vi "4155C PulsedStressV Config SMUs v2.0.vi"(0 "VISA resource name in":refnum<visa-resource-name>, 1 "Pulse period":dbl=0.05 min=0.005 max=1.0 step=0.0001 format="%.4f", 2 "Pulsed Stress V - Source/Common":u32(ring) items=["SMU1  ", "SMU2  ", "SMU3  ", "SMU4  ", "SMU5  ", "SMU6  "], 3 "Pulse width":dbl=0.0005 min=0.0005 max=0.1 step=0.0001 format="%.4f", 4 "Pulsed Stress V - Drain":u32(ring)=1 items=["SMU1  ", "SMU2  ", "SMU3  ", "SMU4  ", "SMU5  ", "SMU6  "], 5 "error in (no error)":errorcluster, 6 "Gate ON voltage":dbl min=-100.0 max=100.0 step=0.005 format="%.3f", 7 "Drain Voltage":dbl min=-100.0 max=100.0 step=0.005 format="%.3f", 8 "Pulsed Stress V - Gate":u32(ring)=2 items=["SMU1  ", "SMU2  ", "SMU3  ", "SMU4  ", "SMU5  ", "SMU6  "], 9 "Pulsed Stress V - Vextra":u32(ring)=1 items=["VSU1  ", "VSU2  "], 10 "Pulsed Stress V - Probe 4":u32(ring)=3 items=["SMU1  ", "SMU2  ", "SMU3  ", "SMU4  ", "SMU5  ", "SMU6  "], 12 "Gate Standby":bool, 13 "Drain Standby":bool, 15 "Probe 4":cluster{"on/off":bool, "Voltage":dbl} {"Voltage" min=-100.0 max=100.0 format="%.2f"}, 17 "Base voltage":dbl format="%^.4e") -> (14 "VISA Resource Name out":refnum<visa-resource-name>, 19 "error out":errorcluster)   [LabVIEW 2016]
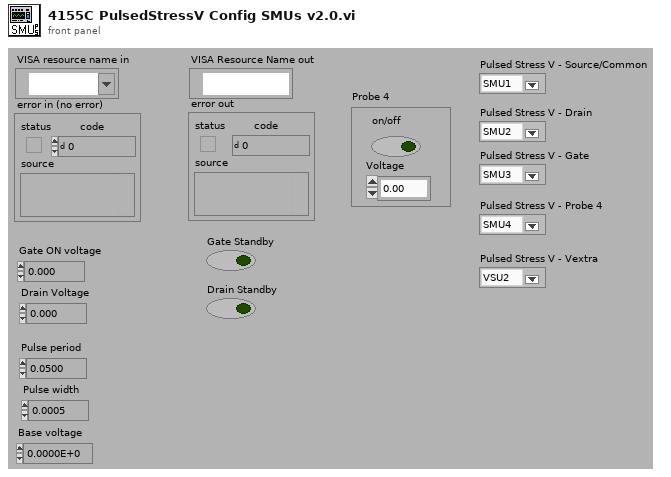
[diagram p1: front panel]
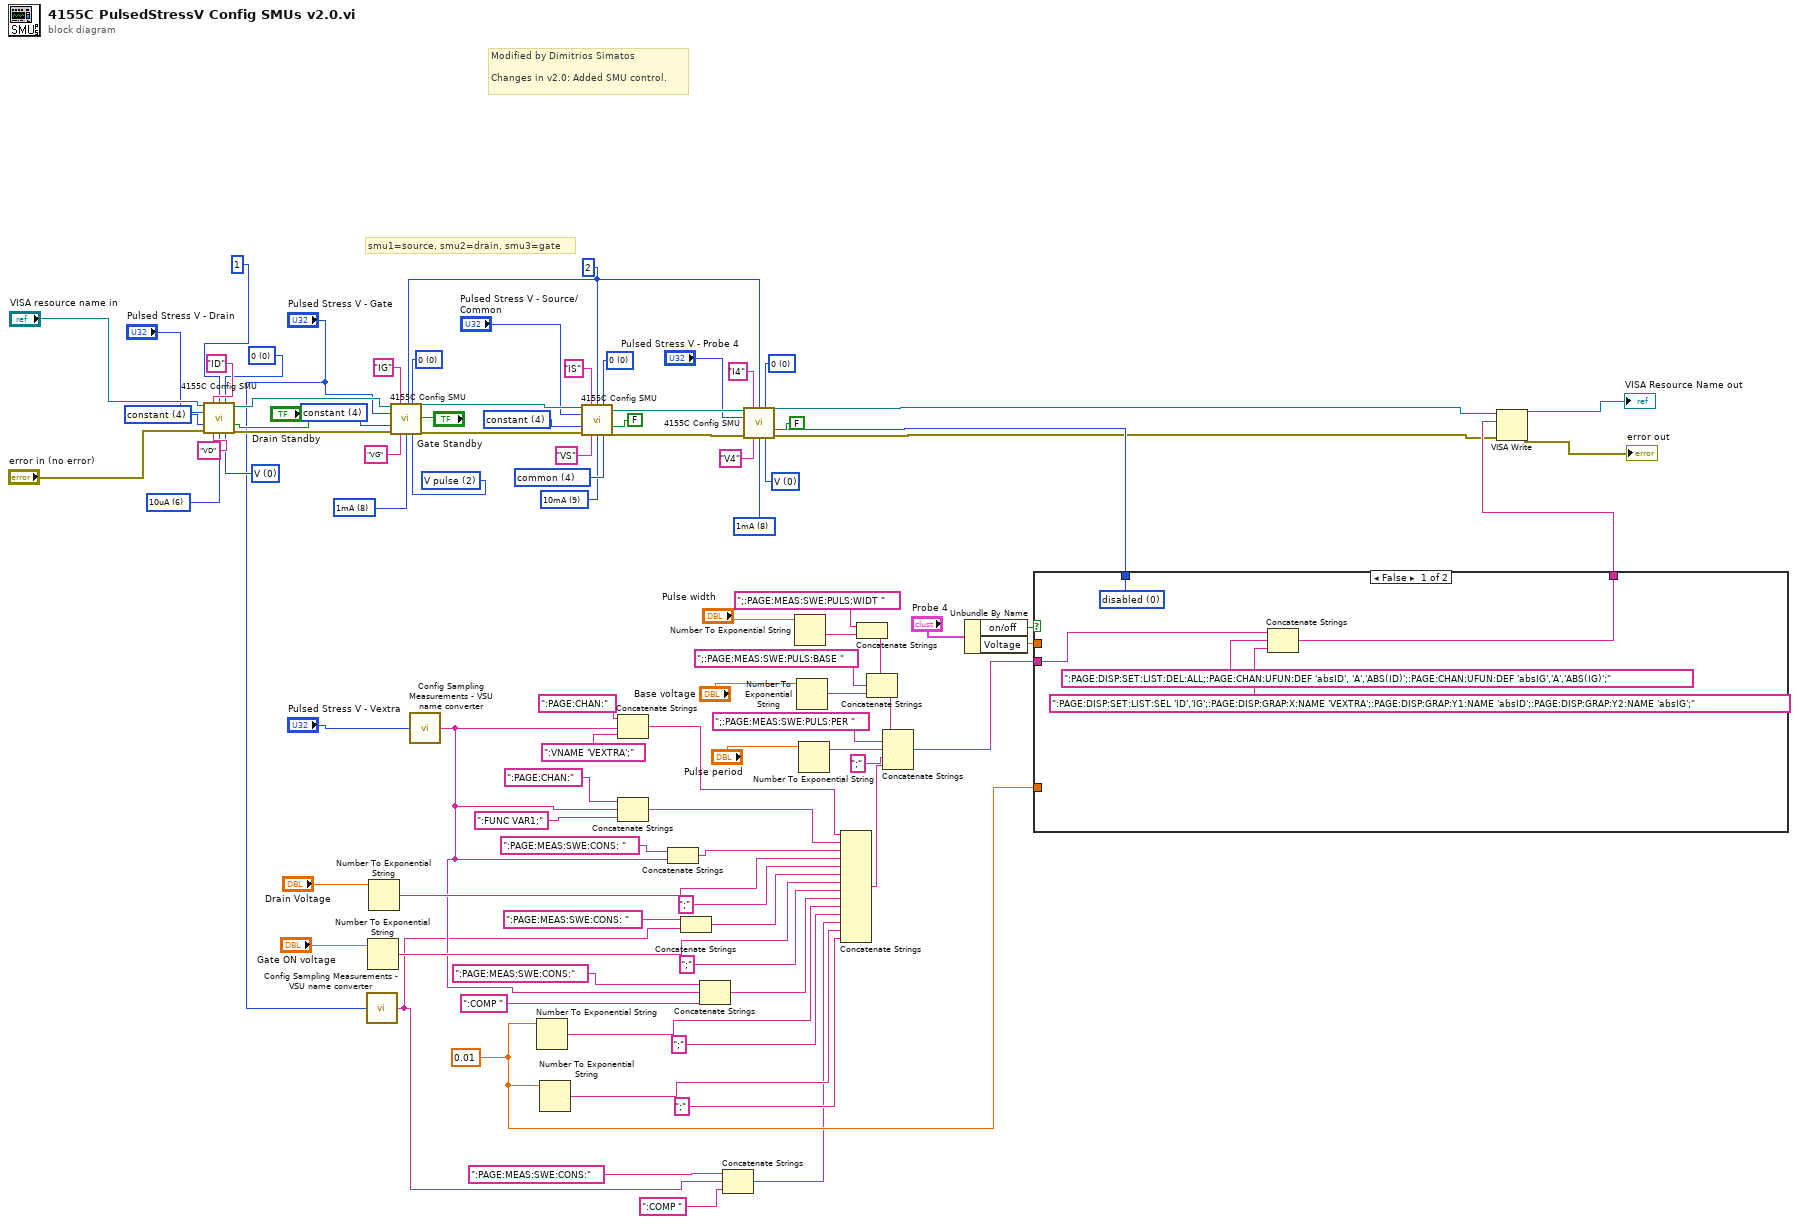
[diagram p0: block diagram]
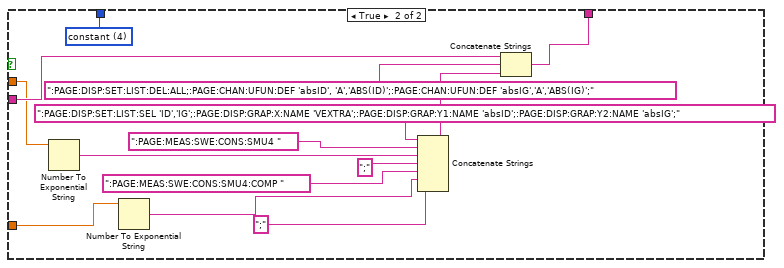
[diagram p2: hidden frame]
diagram:
  w35 = u8 6 items=["10pA  ", "100pA  ", "1nA  ", "10nA", "100nA", "1uA", "10uA", "100uA", "1mA", "10mA", "100mA", "1A"] ("Range")
  w40 = u8 8 items=["10pA  ", "100pA  ", "1nA  ", "10nA", "100nA", "1uA", "10uA", "100uA", "1mA", "10mA", "100mA", "1A"] ("Range")
  w44 = u8 8 items=["10pA  ", "100pA  ", "1nA  ", "10nA", "100nA", "1uA", "10uA", "100uA", "1mA", "10mA", "100mA", "1A"] ("Range")
  w45 = u32 2 items=["V  ", "I  ", "V pulse  ", "I pulse  ", "  common  "] ("mode")
  w43 = 2
  w46 = u8 9 items=["10pA  ", "100pA  ", "1nA  ", "10nA", "100nA", "1uA", "10uA", "100uA", "1mA", "10mA", "100mA", "1A"] ("Range")
  w32 = u32 4 items=["disabled  ", "VAR1  ", "VAR2  ", "VAR1'  ", "constant  "] ("function")
  w29 = u32 0 items=["0  ", "10K Ohms  ", "100K Ohms  ", "1M Ohms  "] ("series resistance *")
  w34 = u32 0 items=["V  ", "I  ", "V pulse  ", "I pulse  ", "  common  "] ("mode")
  w51 = u32 0 items=["V  ", "I  ", "V pulse  ", "I pulse  ", "  common  "] ("mode")
  w52 = u32 0 items=["0  ", "10K Ohms  ", "100K Ohms  ", "1M Ohms  "] ("series resistance *")
  w56 = u32 0 items=["0  ", "10K Ohms  ", "100K Ohms  ", "1M Ohms  "] ("series resistance *")
  w47 = u32 4 items=["disabled  ", "VAR1  ", "VAR2  ", "VAR1'  ", "constant  "] ("function")
  w60 = u32 4 items=["V  ", "I  ", "V pulse  ", "I pulse  ", "  common  "] ("mode")
  w61 = u32 0 items=["0  ", "10K Ohms  ", "100K Ohms  ", "1M Ohms  "] ("series resistance *")
  w63 = u32 4 items=["disabled  ", "VAR1  ", "VAR2  ", "VAR1'  ", "constant  "] ("function")
  w64 = 0.01 ("DRAIN CURRENT compliance")
  # "Modified by Dimitrios Simatos\n\nChanges in v2.0: Added SMU control."
  # "smu1=source, smu2=drain, smu3=gate"
  n1 = call "4155C Config SMU.vi"("VISA session"="VISA resource name in", "I name (max 6 chars)"="ID", "Range mode"=1, "series resistance *"=w29, "unit to configure"="Pulsed Stress V - Drain", "function"=w32, "standby"="Drain Standby", "error in (no error)"="error in (no error)", "V name (max 6 chars)"="VD", "Range"=w35, "mode"=w34) -> ("dup VISA resource name"=w39:refnum<visa-resource-name>, "error out"=w37:errorcluster)  [unwired: 3 in]
  n2 = call "Config Sampling Measurements - VSU name converter.vi"("unit to configure"="Pulsed Stress V - Gate") -> ("VSU to be configured"=w2:string)
  n3 = Number To Exponential String(number="Gate ON voltage") -> (E-format string=w72:string)  [unwired: 3 in]
  n4 = Number To Exponential String(number="Drain Voltage") -> (E-format string=w74:string)  [unwired: 3 in]
  n5 = call "4155C Config SMU.vi"("VISA session"=w39, "I name (max 6 chars)"="IG", "Range mode"=w43, "series resistance *"=w56, "unit to configure"="Pulsed Stress V - Gate", "function"=w47, "standby"="Gate Standby", "error in (no error)"=w37, "V name (max 6 chars)"="VG", "Range"=w44, "mode"=w45) -> ("dup VISA resource name"=w48:refnum<visa-resource-name>, "error out"=w38:errorcluster)  [unwired: 3 in]
  n6 = call "Config Sampling Measurements - VSU name converter.vi"("unit to configure"="Pulsed Stress V - Vextra") -> ("VSU to be configured"=w5:string)
  n7 = Number To Exponential String(number=w64) -> (E-format string=w68:string)  [unwired: 3 in]
  n8 = Number To Exponential String(number=w64) -> (E-format string=w66:string)  [unwired: 3 in]
  n9 = call "4155C Config SMU.vi"("VISA session"=w48, "I name (max 6 chars)"="IS", "Range mode"=w43, "series resistance *"=w61, "unit to configure"="Pulsed Stress V - Source/Common", "function"=w63, "standby"=FALSE, "error in (no error)"=w38, "V name (max 6 chars)"="VS", "Range"=w46, "mode"=w60) -> ("dup VISA resource name"=w42:refnum<visa-resource-name>, "error out"=w41:errorcluster)  [unwired: 3 in]
  n10 = Concatenate Strings(":PAGE:CHAN:", w5, ":VNAME 'VEXTRA';") -> (w17:string)
  n11 = Concatenate Strings(":PAGE:CHAN:", w5, ":FUNC VAR1;") -> (w16:string)
  n12 = Concatenate Strings(":PAGE:MEAS:SWE:CONS: " ("write buffer (\"\")"), w5) -> (w12:string)
  n13 = Concatenate Strings(":PAGE:MEAS:SWE:CONS: " ("write buffer (\"\")"), w2) -> (w10:string)
  n14 = Concatenate Strings(":PAGE:MEAS:SWE:CONS:", w5, ":COMP ") -> (w8:string)
  n15 = Concatenate Strings(":PAGE:MEAS:SWE:CONS:", w2, ":COMP ") -> (w3:string)
  n16 = Number To Exponential String(number="Pulse width") -> (E-format string=w85:string)  [unwired: 3 in]
  n17 = Number To Exponential String(number="Base voltage") -> (E-format string=w81:string)  [unwired: 3 in]
  n18 = Number To Exponential String(number="Pulse period") -> (E-format string=w78:string)  [unwired: 3 in]
  n19 = Concatenate Strings(w17, w16, w12, w74, ";" ("Substring"), w10, w72, ";" ("Substring"), w8, w68, ";" ("Substring"), w3, w66, ";" ("Substring")) -> (w75:string)
  n20 = Concatenate Strings(";:PAGE:MEAS:SWE:PULS:WIDT " ("Substring"), w85) -> (w83:string)
  n21 = Concatenate Strings(w83, ";:PAGE:MEAS:SWE:PULS:BASE " ("Substring"), w81) -> (w79:string)
  n22 = Concatenate Strings(w79, ";:PAGE:MEAS:SWE:PULS:PER " ("Substring"), w78, ";" ("Substring"), w75) -> (w76:string)
  n23 = Unbundle By Name("Probe 4") -> ("on/off"=w91:bool, "Voltage"=w92:dbl)
  n24 = case shown="False" w91 {
    tunnel: w76 -> [w99 w113]
    tunnel: [w98 w112] -> w89
    tunnel: w92 -> [_ w110]
    tunnel: [w97 w111] -> w25
    tunnel: w64 -> [_ w102]
    frame False {
      w97 = u32 0 items=["disabled  ", "VAR1  ", "VAR2  ", "VAR1'  ", "constant  "] ("function")
      n25 = Concatenate Strings(w99, ":PAGE:DISP:SET:LIST:DEL:ALL;:PAGE:CHAN:UFUN:DEF 'absID', 'A','ABS(ID)';:PAGE:CHAN:UFUN:DEF 'absIG','A','ABS(IG)';", ":PAGE:DISP:SET:LIST:SEL 'ID','IG';:PAGE:DISP:GRAP:X:NAME 'VEXTRA';:PAGE:DISP:GRAP:Y1:NAME 'absID';:PAGE:DISP:GRAP:Y2:NAME 'absIG';" ("write buffer (\"\")")) -> (w98:string)
    }
    frame True {
      w111 = u32 4 items=["disabled  ", "VAR1  ", "VAR2  ", "VAR1'  ", "constant  "] ("function")
      n26 = Number To Exponential String(number=w110) -> (E-format string=w108:string)  [unwired: 3 in]
      n27 = Number To Exponential String(number=w102) -> (E-format string=w104:string)  [unwired: 3 in]
      n28 = Concatenate Strings(":PAGE:DISP:SET:LIST:SEL 'ID','IG';:PAGE:DISP:GRAP:X:NAME 'VEXTRA';:PAGE:DISP:GRAP:Y1:NAME 'absID';:PAGE:DISP:GRAP:Y2:NAME 'absIG';" ("write buffer (\"\")"), ":PAGE:MEAS:SWE:CONS:SMU4 " ("write buffer (\"\")"), w108, ";" ("Substring"), ":PAGE:MEAS:SWE:CONS:SMU4:COMP ", w104, ";" ("Substring")) -> (w100:string)
      n29 = Concatenate Strings(w113, ":PAGE:DISP:SET:LIST:DEL:ALL;:PAGE:CHAN:UFUN:DEF 'absID', 'A','ABS(ID)';:PAGE:CHAN:UFUN:DEF 'absIG','A','ABS(IG)';", w100) -> (w112:string)
    }
  }
  n30 = call "4155C Config SMU.vi"("VISA session"=w42, "I name (max 6 chars)"="I4", "Range mode"=w43, "series resistance *"=w52, "unit to configure"="Pulsed Stress V - Probe 4", "function"=w25, "standby"=FALSE, "error in (no error)"=w41, "V name (max 6 chars)"="V4", "Range"=w40, "mode"=w51) -> ("dup VISA resource name"=w26:refnum<visa-resource-name>, "error out"=w24:errorcluster)  [unwired: 3 in]
  n31 = VISA Write(VISA resource name=w26, write buffer=w89, error in (no error)=w24) -> (VISA resource name out=→"VISA Resource Name out":refnum<visa-resource-name>, error out=→"error out":errorcluster)  [unwired: 1 out]
